vi "TestArraytoWave.vi"(8 "error in (no error)":errorcluster) -> (0 "error out":errorcluster)   [LabVIEW 2019]
uses:
  private/Igor_NumericArraytoIgorWave.vi
  private/Igor_StringArraytoIgorWave.vi
  <vilib>/addons/_JKI Toolkits/Caraya/classes/Test/Test.lvclass
  <vilib>/addons/_JKI Toolkits/Caraya/classes/Assert/Assert.lvclass
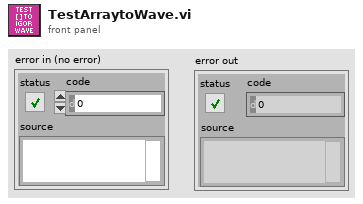
[diagram p1: front panel]
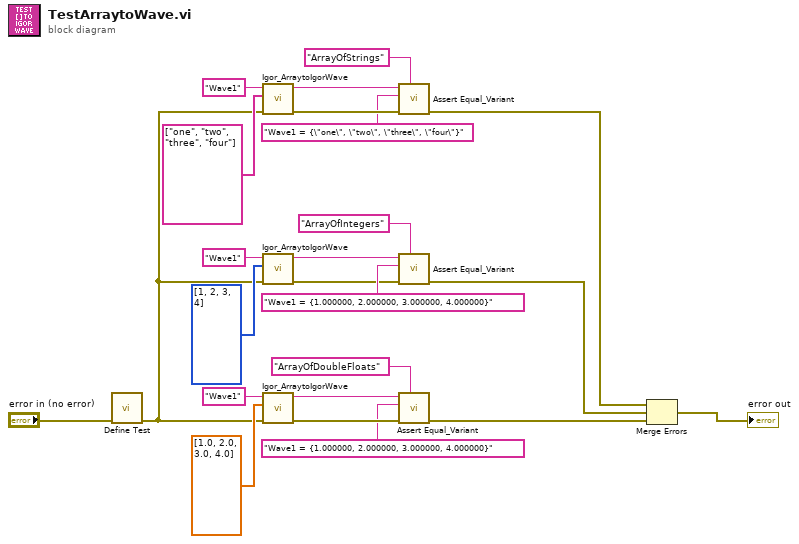
[diagram p0: block diagram]
diagram:
  n1 = call <vilib>:"Define Test.vi"("error in (no error)"="error in (no error)") -> ("error out"=w1:errorcluster)  [unwired: 10 in]
  n2 = call-poly "Igor_ArraytoIgorWave.vi"("error in (no error)"=w1, "Wave"=string[] ["one", "two", "three", "four"], "Name"="Wave1") -> ("error out"=w7:errorcluster, "Igor Wave"=w6:string)  [unwired: 7 in]
  n3 = call-poly "Igor_ArraytoIgorWave.vi"("error in (no error)"=w1, "Wave"=i32[] [1, 2, 3, 4], "Name"="Wave1") -> ("error out"=w12:errorcluster, "Igor Wave"=w13:string)  [unwired: 7 in]
  n4 = call-poly "Igor_ArraytoIgorWave.vi"("error in (no error)"=w1, "Wave"=dbl[] [1.0, 2.0, 3.0, 4.0], "Name"="Wave1") -> ("error out"=w20:errorcluster, "Igor Wave"=w19:string)  [unwired: 7 in]
  n5 = call <vilib>:"Assert Equal_Variant.vi"("Label"="ArrayOfStrings", "error in (no error)"=w7, "Y"="Wave1 = {\"one\", \"two\", \"three\", \"four\"}", "X"=w6) -> ("error out"=w2:errorcluster)  [unwired: 7 in]
  n6 = call <vilib>:"Assert Equal_Variant.vi"("Label"="ArrayOfIntegers", "error in (no error)"=w12, "Y"="Wave1 = {1.000000, 2.000000, 3.000000, 4.000000}", "X"=w13) -> ("error out"=w10:errorcluster)  [unwired: 7 in]
  n7 = call <vilib>:"Assert Equal_Variant.vi"("Label"="ArrayOfDoubleFloats", "error in (no error)"=w20, "Y"="Wave1 = {1.000000, 2.000000, 3.000000, 4.000000}", "X"=w19) -> ("error out"=w22:errorcluster)  [unwired: 7 in]
  n8 = Merge Errors(w2, w10, w22) -> (→"error out":errorcluster)
